vi "Read_Key_Database.vi"(11 "configuration file path":path) -> (2 "key values":string[](array[string]), 3 "key names":string[](array[string]))   [LabVIEW 2023, in "LP_CRC.lvlib"]
uses:
  LP_CRC.lvlib
  <vilib>/Utility/config.llb/NI_LVConfig.lvlib
  <vilib>/Utility/config.llb/Read Key (String).vi
panel:
  out "size(s)":i32
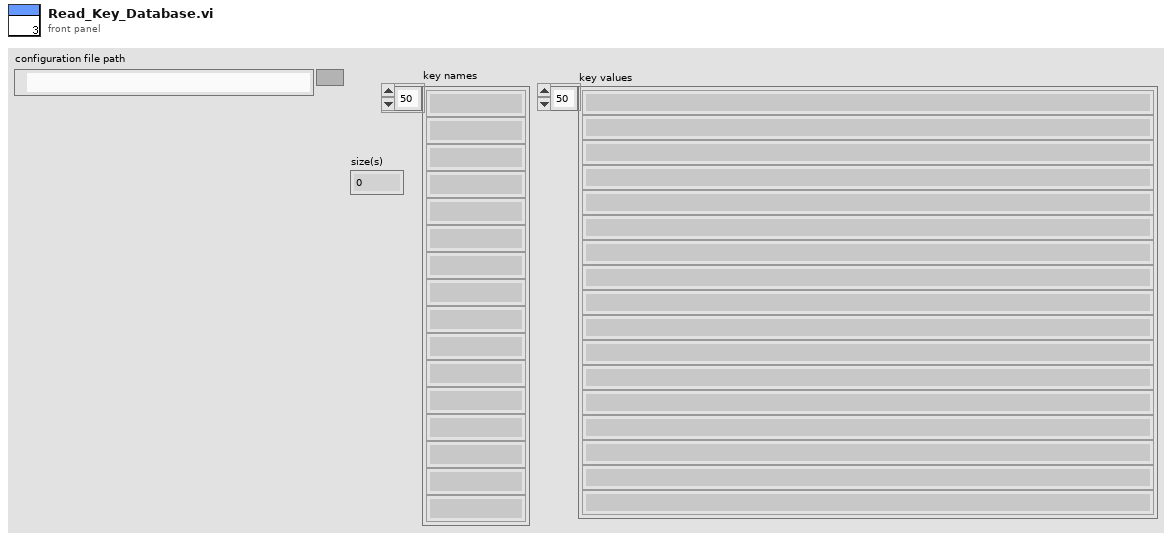
[diagram p1: front panel]
types:
  T1 = typedef "NI_LVConfig.lvlib/Config Data RefNum.ctl" = refnum<k1>
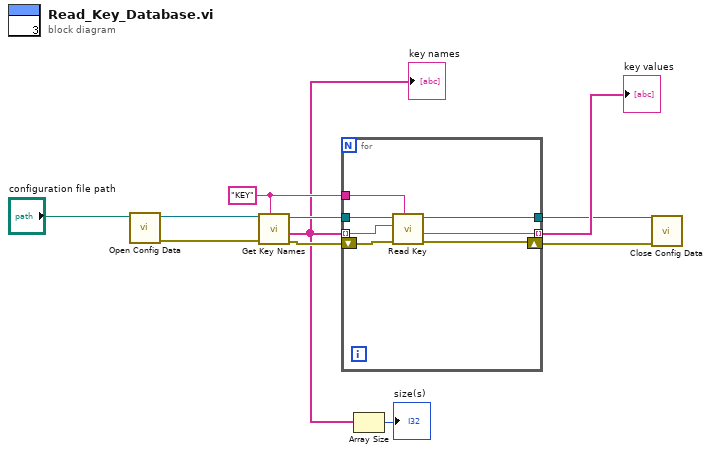
[diagram p0: block diagram]
diagram:
  w8 = "KEY" ("section")
  n1 = call <vilib>:"Open Config Data.vi"("configuration file path"="configuration file path") -> ("error out"=w10:errorcluster, "refnum"=w11:T1)  [unwired: 8 in, 1 out]
  n2 = call <vilib>:"Get Key Names.vi"("section"=w8, "error in (no error)"=w10, "refnum"=w11) -> ("error out"=w7:errorcluster, "key names"=w2:string[], "refnum out"=w9:T1)  [unwired: 5 in, 1 out]
  "key names" <- w2
  n3 = for {
    tunnel: w9 -> [w18]
    tunnel: w8 -> [w17]
    tunnel: w2 -> [w16] mode=indexing
    shift-right: [w14] -> w5
    shift-left: w7 -> [w15]
    tunnel: [w13] -> w6 mode=indexing
    tunnel: [w12] -> w4
    n4 = call-poly <vilib>:"Read Key.vi"("section"=w17, "error in (no error)"=w15, "key"=w16, "refnum"=w18) -> ("error out"=w14:errorcluster, "value"=w13:string, "refnum out"=w12:T1)  [unwired: 4 in, 1 out]
  }
  "key values" <- w6
  n5 = Array Size(array=w2) -> (size(s)=→"size(s)":i32)
  n6 = call <vilib>:"Close Config Data.vi"("error in (no error)"=w5, "refnum"=w4) -> ()  [unwired: 8 in, 2 out]
